vi "Get Current.vi"(8 "error in (no error)":errorcluster, 10 "Tree name":string, 11 "Tree in":refnum<class "Tree.lvclass">) -> (0 "error out":errorcluster, 2 "Current shot out":i32, 3 "Tree out":refnum<class "Tree.lvclass">)   [LabVIEW 2012, in "MDSplus.lvlib" / "Tree.lvclass"]
doc: "Return the current shot for that tree."
uses:
  <vilib>/MDSplus/Classes/Tree_Class/Tree.lvclass
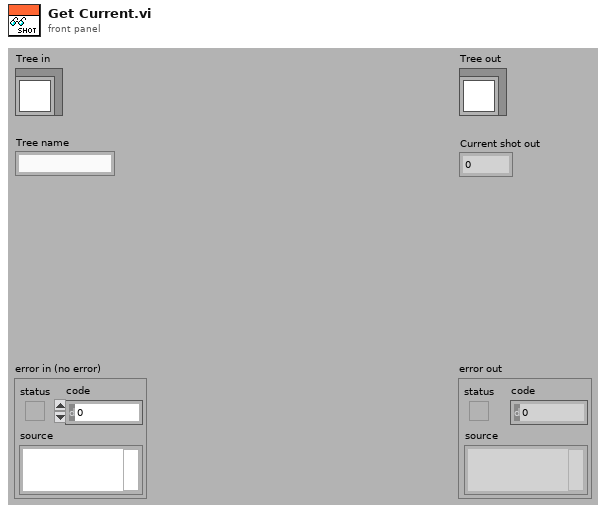
[diagram p1: front panel]
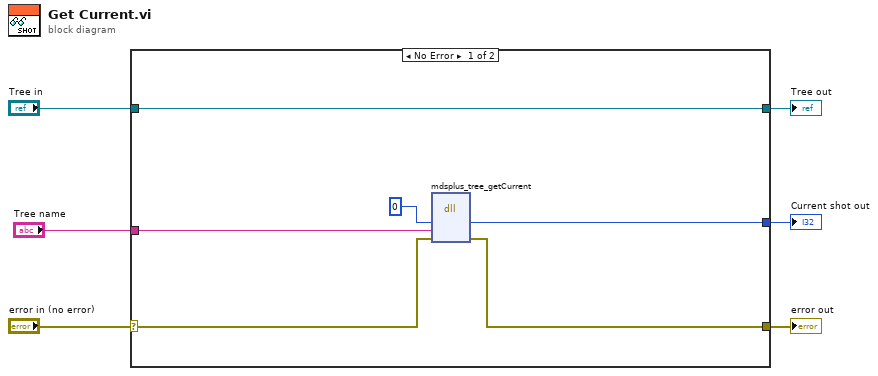
[diagram p0: block diagram]
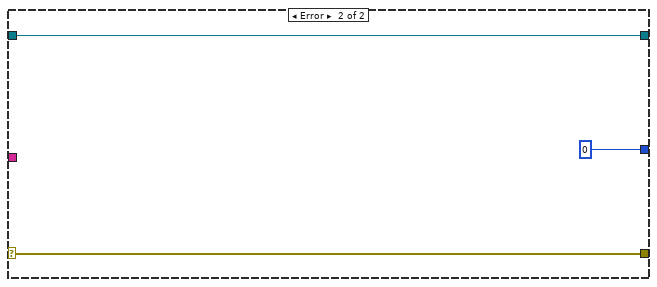
[diagram p2: hidden frame]
diagram:
  n1 = case shown="No Error" "error in (no error)" {
    selector: "error in (no error)" -> [w11 w15]
    tunnel: [w10 w15] -> w5
    tunnel: [w8 w14] -> w3
    tunnel: "Tree in" -> [w8 w14]
    tunnel: [w12 0 ("size")] -> w2
    tunnel: "Tree name" -> [w7 _]
    frame No Error {
      n2 = dll-call lib="MDSobjectsLVShr" fn="mdsplus_tree_getCurrent"("currentOut"=0 ("size"), "treeNameIn"=w7, "error"=w11) -> ("currentOut"=w12:i32, "error"=w10:errorcluster)  [unwired: 5 in, 2 out]
    }
    frame Error {
    }
  }
  "error out" <- w5
  "Tree out" <- w3
  "Current shot out" <- w2
